vi "intersect line.vi"(1 "R pos":dbl[](array[numeric])=[0.0, 0.0], 2 "max dist":dbl=40.0, 3 "look dir":dbl(slide) scale=3.2..-3.2, 4 "P2y":dbl[](array[numeric])=[-15.0, -15.0], 5 "P2x":dbl[](array[numeric])=[10.0, 20.0], 6 "P1y":dbl[](array[numeric])=[15.0, 20.0], 7 "P1x":dbl[](array[numeric])) -> (0 "Dist":dbl)   [LabVIEW 2009]
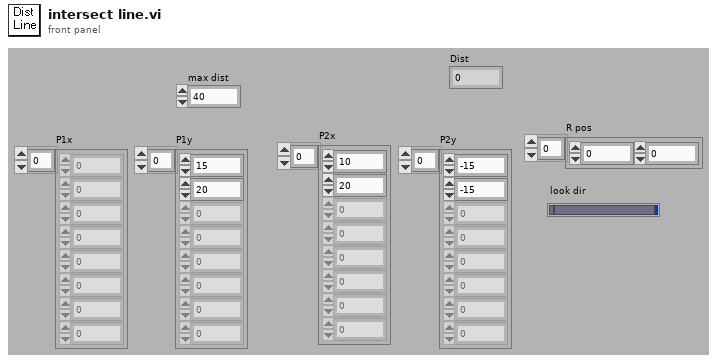
[diagram p1: front panel]
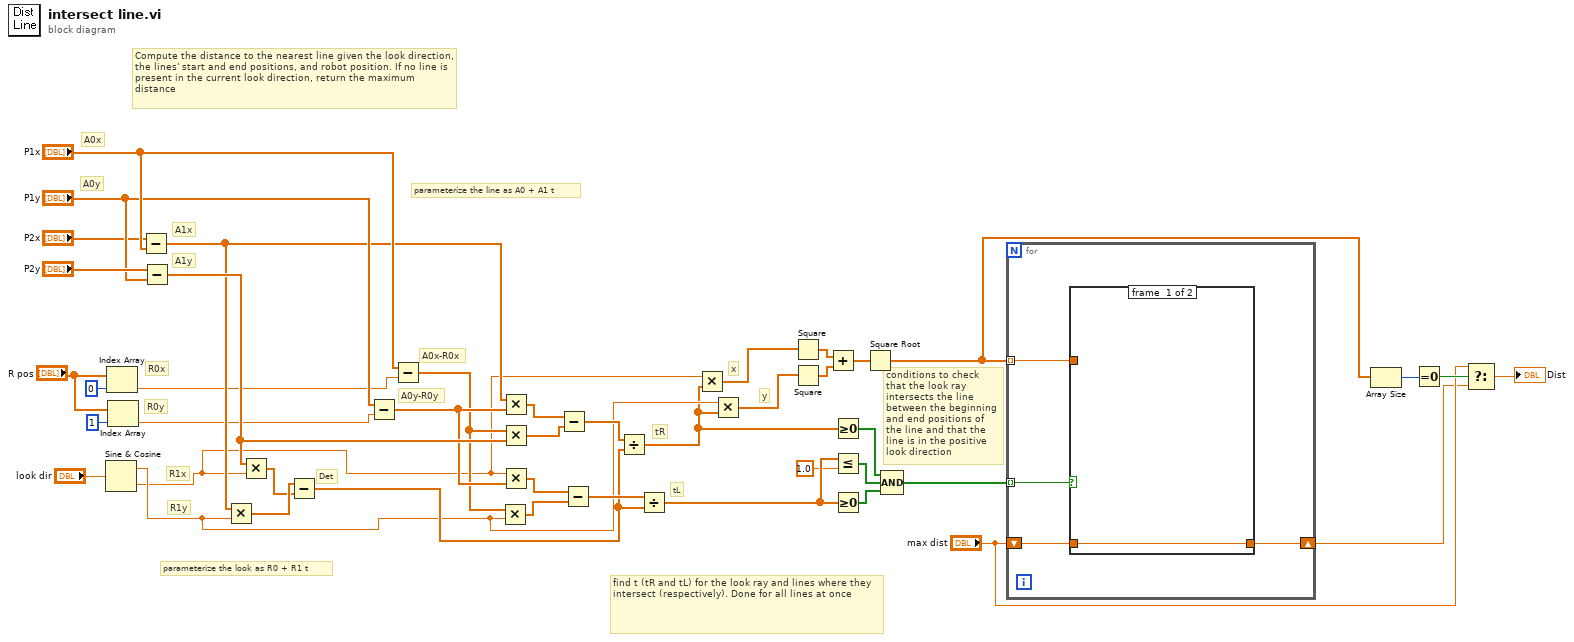
[diagram p0: block diagram]
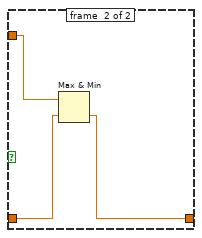
[diagram p2: hidden frame]
diagram:
  # "conditions to check that the look ray intersects the line between the beginning and end positions of the line and that the line is in the positive look direction"
  # "find t (tR and tL) for the look ray and lines where they intersect (respectively). Done for all lines at once"
  # "parameterize the look as R0 + R1 t"
  # "parameterize the line as A0 + A1 t"
  # "Compute the distance to the nearest line given the look direction, the lines' start and end positions, and robot position. If no line is present in the current look direction, return the maximum distance"
  # "y"
  # "x"
  # "tL"
  # "tR"
  # "A0y-R0y"
  # "A0x-R0x"
  # "Det"
  # "R1y"
  # "R1x"
  # "R0y"
  # "R0x"
  # "A1y"
  # "A1x"
  # "A0y"
  # "A0x"
  n1 = Sine & Cosine(0:"look dir") -> (1:w13:dbl, 2:w12:dbl)
  n2 = Index Array(array="R pos", index=0) -> (element=w7:dbl)
  n3 = Index Array(array="R pos", index=1) -> (element=w20:dbl)
  n4 = Subtract(x="P2x", y="P1x") -> (x-y=w24:dbl[])
  n5 = Subtract(x="P2y", y="P1y") -> (x-y=w37:dbl[])
  n6 = Multiply(x=w24, y=w13) -> (x*y=w39:dbl[])
  n7 = Multiply(x=w37, y=w12) -> (x*y=w38:dbl[])
  n8 = Subtract(x=w39, y=w38) -> (x-y=w28:dbl[])
  n9 = Subtract(x="P1y", y=w20) -> (x-y=w34:dbl[])
  n10 = Subtract(x="P1x", y=w7) -> (x-y=w33:dbl[])
  n11 = Multiply(x=w33, y=w13) -> (x*y=w31:dbl[])
  n12 = Multiply(x=w24, y=w34) -> (x*y=w36:dbl[])
  n13 = Multiply(x=w33, y=w37) -> (x*y=w35:dbl[])
  n14 = Multiply(x=w12, y=w34) -> (x*y=w32:dbl[])
  n15 = Subtract(x=w36, y=w35) -> (x-y=w30:dbl[])
  n16 = Subtract(x=w32, y=w31) -> (x-y=w29:dbl[])
  n17 = Divide(x=w30, y=w28) -> (x/y=w11:dbl[])
  n18 = Divide(x=w29, y=w28) -> (x/y=w23:dbl[])
  n19 = Multiply(x=w12, y=w11) -> (x*y=w8:dbl[])
  n20 = Multiply(x=w13, y=w11) -> (x*y=w9:dbl[])
  n21 = Square(x=w8) -> (x^2=w18:dbl[])
  n22 = Square(x=w9) -> (x^2=w17:dbl[])
  n23 = Add(x=w18, y=w17) -> (x+y=w16:dbl[])
  n24 = Greater Or Equal To 0?(x=w11) -> (x >= 0?=w10:bool[])
  n25 = Less Or Equal?(x=w23, y=1.0) -> (x <= y?=w22:bool[])
  n26 = Greater Or Equal To 0?(x=w23) -> (x >= 0?=w21:bool[])
  n27 = Square Root(x=w16) -> (sqrt(x)=w6:dbl[])
  n28 = Compound Arithmetic op=AND(w10, w22, w21) -> (w19:bool[])
  n29 = for {
    tunnel: w19 -> [w47] mode=indexing
    shift-right: [w45] -> w2
    shift-left: "max dist" -> [w46]
    tunnel: w6 -> [w44] mode=indexing
    n30 = case shown="True" w47 {
      tunnel: w46 -> [w48 w50]
      tunnel: [w48 w49] -> w45
      tunnel: w44 -> [_ w51]
      frame #0 {
      }
      frame #1 {
        n31 = Max & Min(x=w51, y=w50) -> (min(x,y)=w49:dbl)  [unwired: 1 out]
      }
    }
  }
  n32 = Array Size(array=w6) -> (size(s)=w5:i32)
  n33 = Equal To 0?(x=w5) -> (x = 0?=w4:bool)
  n34 = Select(t="max dist", s=w4, f=w2) -> (s? t:f=→"Dist":dbl)
